vi "Simulation-2 (For loop-square)_B220061.vi"() -> ()   [LabVIEW 2021]
panel:
  out "Array of Squares":i32[](array[numeric])
  out "x^2":i32
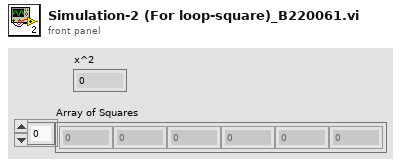
[diagram p1: front panel]
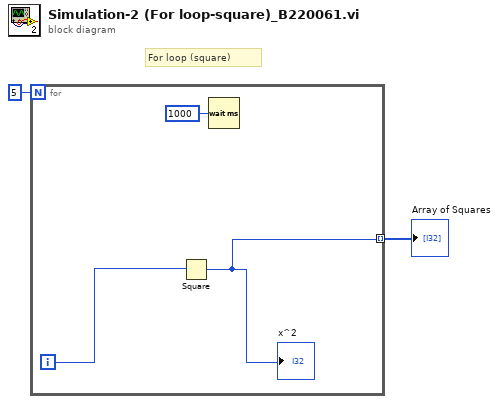
[diagram p0: block diagram]
diagram:
  # "For loop (square)"
  n1 = for {
    N: 5 -> [_]
    tunnel: [w3] -> w2 mode=indexing
    i -> [w4]
    n2 = Square(x=w4) -> (x^2=w3:i32)
    "x^2" <- w3
    n3 = Wait (ms)(milliseconds to wait=u32 1000) -> ()  [unwired: 1 out]
  }
  "Array of Squares" <- w2
